vi "TRAJECTORY_EXECUTE_SWERVE.vi"(4 "Time Offset":dbl=-1.0 format="%16.4f", 6 "EnableClosedLoop":bool=TRUE, 8 "Init":bool, 9 "Reverse":bool, 10 "Follow Orientation":bool, 11 "Gyro Heading\nRAD":dbl) -> (0 "AtReference":bool, 1 "OutputTRAJ_STATE":T6={"TimeSeconds"=0.0, "Velocity"=0.0, "Acceleration"=0.0, "POSE"={"TRANSLATION"={"X"=0.0, "Y"=0.0}, "ROTATION"={"VALUE"=0.0, "COS"=1.0, "SIN"=0.0}}, "Curvature"=0.0} {"POSE"."ROTATION"."SIN" format="%13.4f"; "POSE"."ROTATION"."COS" format="%13.4f"; "POSE"."ROTATION"."VALUE" format="%13.4f"; "POSE"."TRANSLATION"."Y" format="%14.3f"; "POSE"."TRANSLATION"."X" format="%14.3f"}, 2 "Error and Corr":T4 {"Error Pose"."ROTATION"."SIN" format="%13.4f"; "Error Pose"."ROTATION"."COS" format="%13.4f"; "Error Pose"."ROTATION"."VALUE" format="%13.4f"; "Error Pose"."TRANSLATION"."Y" format="%14.3f"; "Error Pose"."TRANSLATION"."X" format="%14.3f"}, 3 "Chassis Velocity Target":T5 {"vOmega" format="%10.3f"; "vY" format="%10.3f"; "vX" format="%10.3f"}, 5 "Orientation Target":dbl)   [LabVIEW 2019]
uses:
  <vilib>/Rock Robotics/WPI/ThirdParty/JAS_Junk/TrajLib/TRAJ_STATE.ctl
  <vilib>/Rock Robotics/WPI/ThirdParty/JAS_Junk/TrajLib/POSE2D.ctl
  <vilib>/Rock Robotics/WPI/ThirdParty/JAS_Junk/TrajLib/TRANSLATION2D.ctl
  <vilib>/Rock Robotics/WPI/ThirdParty/JAS_Junk/TrajLib/ROTATION2D.ctl
  <vilib>/Rock Robotics/WPI/ThirdParty/JAS_Junk/TrajLib/CHASSIS_SPEEDS.ctl
  <vilib>/Rock Robotics/WPI/ThirdParty/JAS_Junk/TrajLib/Translation_Create.vi
  <vilib>/Rock Robotics/WPI/ThirdParty/JAS_Junk/TrajLib/ProfiledPIDController_NewPeriod.vi
  <vilib>/Rock Robotics/WPI/ThirdParty/JAS_Junk/TrajLib/PIDController_NewPeriod.vi
  <vilib>/Rock Robotics/WPI/ThirdParty/JAS_Junk/TrajLib/MathUtil_InputModulus.vi
  <vilib>/Rock Robotics/WPI/ThirdParty/JAS_Junk/TrajLib/Rotation_UnaryMinus.vi
  <vilib>/Rock Robotics/WPI/ThirdParty/JAS_Junk/TrajLib/Rotation_RotateBy.vi
  <vilib>/Rock Robotics/WPI/ThirdParty/JAS_Junk/TrajLib/HolDrvCtrl_Calculate.vi
  <vilib>/Rock Robotics/WPI/ThirdParty/JAS_Junk/TrajLib/Pose_getXYAngle.vi
  <vilib>/Rock Robotics/WPI/ThirdParty/JAS_Junk/TrajLib/TrapProfState_New.vi
  <vilib>/Rock Robotics/SystemInterfaces/NetworkCommunication/NetComm_UsageReport_report.vi
  <vilib>/Rock Robotics/WPI/ThirdParty/JAS_Junk/TrajLib/Rotation_CreateXY.vi
  <vilib>/Rock Robotics/WPI/ThirdParty/JAS_Junk/TrajLib/ProfiledPIDController_Calculate_Meas_Goal.vi
  <vilib>/Rock Robotics/WPI/ThirdParty/JAS_Junk/TrajLib/ChassisSpeeds_FromFieldRelativeSpeeds.vi
  <vilib>/Rock Robotics/WPI/ThirdParty/JAS_Junk/TrajLib/PIDController_Reset.vi
  <vilib>/Rock Robotics/WPI/ThirdParty/JAS_Junk/TrajLib/PIDController_Calculate_SP_PV.vi
  <vilib>/Rock Robotics/WPI/ThirdParty/JAS_Junk/TrajLib/ProfiledPIDController_Reset_PosOnly.vi
  <vilib>/Rock Robotics/WPI/ThirdParty/JAS_Junk/TrajLib/Rotation_GetAngleCosSin.vi
  <vilib>/Rock Robotics/WPI/ThirdParty/JAS_Junk/TrajLib/Pose_RelativeTo.vi
  <vilib>/Rock Robotics/WPI/ThirdParty/JAS_Junk/TrajLib/Util_CalcDist.vi
  <vilib>/Rock Robotics/WPI/ThirdParty/JAS_Junk/TrajLib/ProfiledPIDController_SetGoal_PosOnly.vi
  <vilib>/Rock Robotics/WPI/ThirdParty/JAS_Junk/TrajLib/ProfiledPIDController_Calculate_Meas.vi
  <vilib>/Rock Robotics/WPI/ThirdParty/JAS_Junk/TrajLib/Rotation_GetCos.vi
  <vilib>/Rock Robotics/WPI/ThirdParty/JAS_Junk/TrajLib/Rotation_GetSin.vi
  <vilib>/Rock Robotics/WPI/ThirdParty/JAS_Junk/TrajLib/PIDController_SetSetpoint.vi
  <vilib>/Rock Robotics/WPI/ThirdParty/JAS_Junk/TrajLib/PIDController_Calculate_PV.vi
  <vilib>/Rock Robotics/WPI/ThirdParty/JAS_Junk/TrajLib/ProfiledPIDController_Reset.vi
  <vilib>/Rock Robotics/WPI/ThirdParty/JAS_Junk/TrajLib/Transform_Create_PosePose.vi
  <vilib>/Rock Robotics/WPI/ThirdParty/JAS_Junk/TrajLib/ProfiledPIDController_SetGoal.vi
  <vilib>/Rock Robotics/WPI/ThirdParty/JAS_Junk/TrajLib/TrapProfile_New.vi
  <vilib>/Rock Robotics/WPI/ThirdParty/JAS_Junk/TrajLib/ProfiledPIDController_GetPeriod.vi
  <vilib>/Rock Robotics/WPI/ThirdParty/JAS_Junk/TrajLib/TrapProfile_Calculate.vi
  <vilib>/Rock Robotics/WPI/ThirdParty/JAS_Junk/TrajLib/ControllerUtil_GetModulusError.vi
  <vilib>/Rock Robotics/WPI/ThirdParty/JAS_Junk/TrajLib/Translation_RotateBy.vi
  <vilib>/Rock Robotics/WPI/ThirdParty/JAS_Junk/TrajLib/Translation_Minus.vi
  <vilib>/Rock Robotics/WPI/ThirdParty/JAS_Junk/TrajLib/TrapProfile_ShouldFlipAcceleration.vi
  <vilib>/Rock Robotics/WPI/ThirdParty/JAS_Junk/TrajLib/TrapProfile_Direct.vi
  <vilib>/Rock Robotics/WPI/ThirdParty/JAS_Junk/TrajLib/PIDController_GetPeriod.vi
  <vilib>/Rock Robotics/WPI/ThirdParty/JAS_Junk/TrajLib/Util_LibraryGlobals.vi
  <vilib>/Rock Robotics/WPI/ThirdParty/JAS_Junk/TrajLib/Trajectory_Library.lvlib
panel:
  # "(FOR TESTING)"
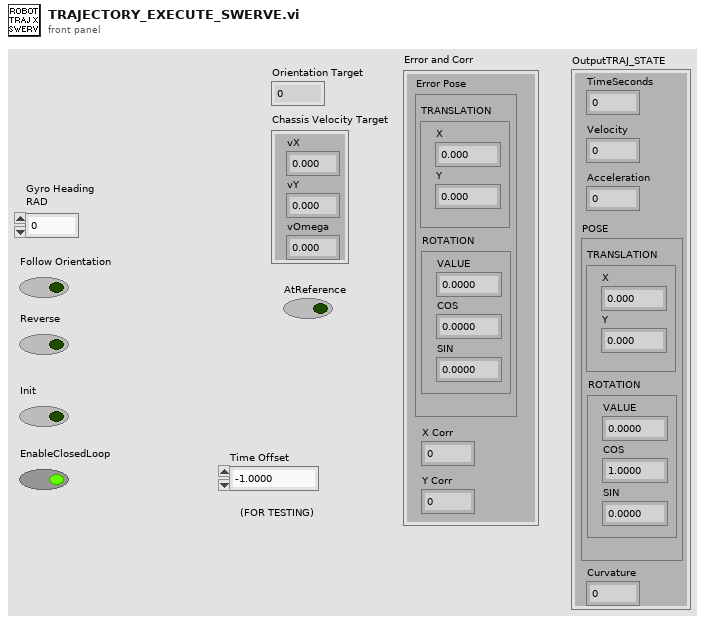
[diagram p1: front panel]
types:
  T1 = typedef "Trajectory_Library.lvlib/POSE2D.ctl" = cluster{"TRANSLATION":T2, "ROTATION":T3}
  T2 = typedef "Trajectory_Library.lvlib/TRANSLATION2D.ctl" = cluster{"X":dbl, "Y":dbl}
  T3 = typedef "Trajectory_Library.lvlib/ROTATION2D.ctl" = cluster{"VALUE":dbl, "COS":dbl, "SIN":dbl}
  T4 = cluster{"Error Pose":T1, "X Corr":dbl, "Y Corr":dbl}
  T5 = typedef "Trajectory_Library.lvlib/CHASSIS_SPEEDS.ctl" = cluster{"vX":dbl, "vY":dbl, "vOmega":dbl}
  T6 = typedef "Trajectory_Library.lvlib/TRAJ_STATE.ctl" = cluster{"TimeSeconds":dbl, "Velocity":dbl, "Acceleration":dbl, "POSE":T1, "Curvature":dbl}
  T7 = typedef "Trajectory_Library.lvlib/SWERVE_DRIVE_KINEMATICS.ctl" = cluster{"NumModules":i32, "InverseKinematics":T8, "ForwardKinematics":T8, "Modules":T2[], "PrevCoR":T2}
  T8 = typedef "NI_Matrix.lvlib/RealMatrix.ctl" = dbl[][]
  T9 = typedef "Trajectory_Library.lvlib/SWERVE_DRIVE_ODOMETRY.ctl" = cluster{"POSE":T1, "GyroOffset":T3, "PreviousAngle":T3, "PrevTime":dbl}
  T10 = typedef "Trajectory_Library.lvlib/TRAJECTORY.ctl" = cluster{"TotalTImeSecs":dbl, "States":T6[]}
  T11 = typedef "Trajectory_Library.lvlib/SWERVE_DRIVE_MODULE_STATE.ctl" = cluster{"Speed":dbl, "Angle":T3}
  T12 = typedef "Trajectory_Library.lvlib/PID_TUNING.ctl" = cluster{"Kp":dbl, "Ki":dbl, "Kd":dbl, "MaximumIntegral":dbl, "MinimumIntegral":dbl}
  T13 = typedef "Trajectory_Library.lvlib/PROFILED_PID_CONTROLLER.ctl" = cluster{"Controller":T14, "Goal":T15, "Setpoint":T15, "Constraint":T16}
  T14 = typedef "Trajectory_Library.lvlib/PID_CONTROLLER.ctl" = cluster{"Kp":dbl, "Ki":dbl, "Kd":dbl, "Period":dbl, "Max_Integral":dbl, "Min_Integral":dbl, "Max_Input":dbl, "Min_Input":dbl, "Continuous":bool, "PositionError":dbl, "VelocityError":dbl, "PrevError":dbl, "TotalError":dbl, "PositionTolerance":dbl, "VelocityTolerance":dbl, "SetPoint":dbl, "Kf":dbl, "Prev_Deriv":dbl, "Prev_Deriv 2":dbl, "DerivativeFilter":bool, "Min_Output":dbl, "Max_Output":dbl, "Prev_F_P":dbl, "Prev_F_P_2":dbl, "AntiWindupActive":bool, "Measurement":dbl}
  T15 = typedef "Trajectory_Library.lvlib/TRAPEZOID_PROFILE_STATE.ctl" = cluster{"Position":dbl, "Velocity":dbl}
  T16 = typedef "Trajectory_Library.lvlib/TRAPEZOID_PROFILE_CONSTRAINT.ctl" = cluster{"MaxVelocity":dbl, "MaxAcceleration":dbl}
  T17 = typedef "Trajectory_Library.lvlib/HOLONOMIC_DRV_CTRL.ctl" = cluster{"poseTolerance":T1, "poseError":T1, "Enabled":bool, "PID_xCtrl":T14, "PID_yCtrl":T14, "PROF_PID_thetaCtrl":T13, "RotationError":T3, "FirstRun":bool}
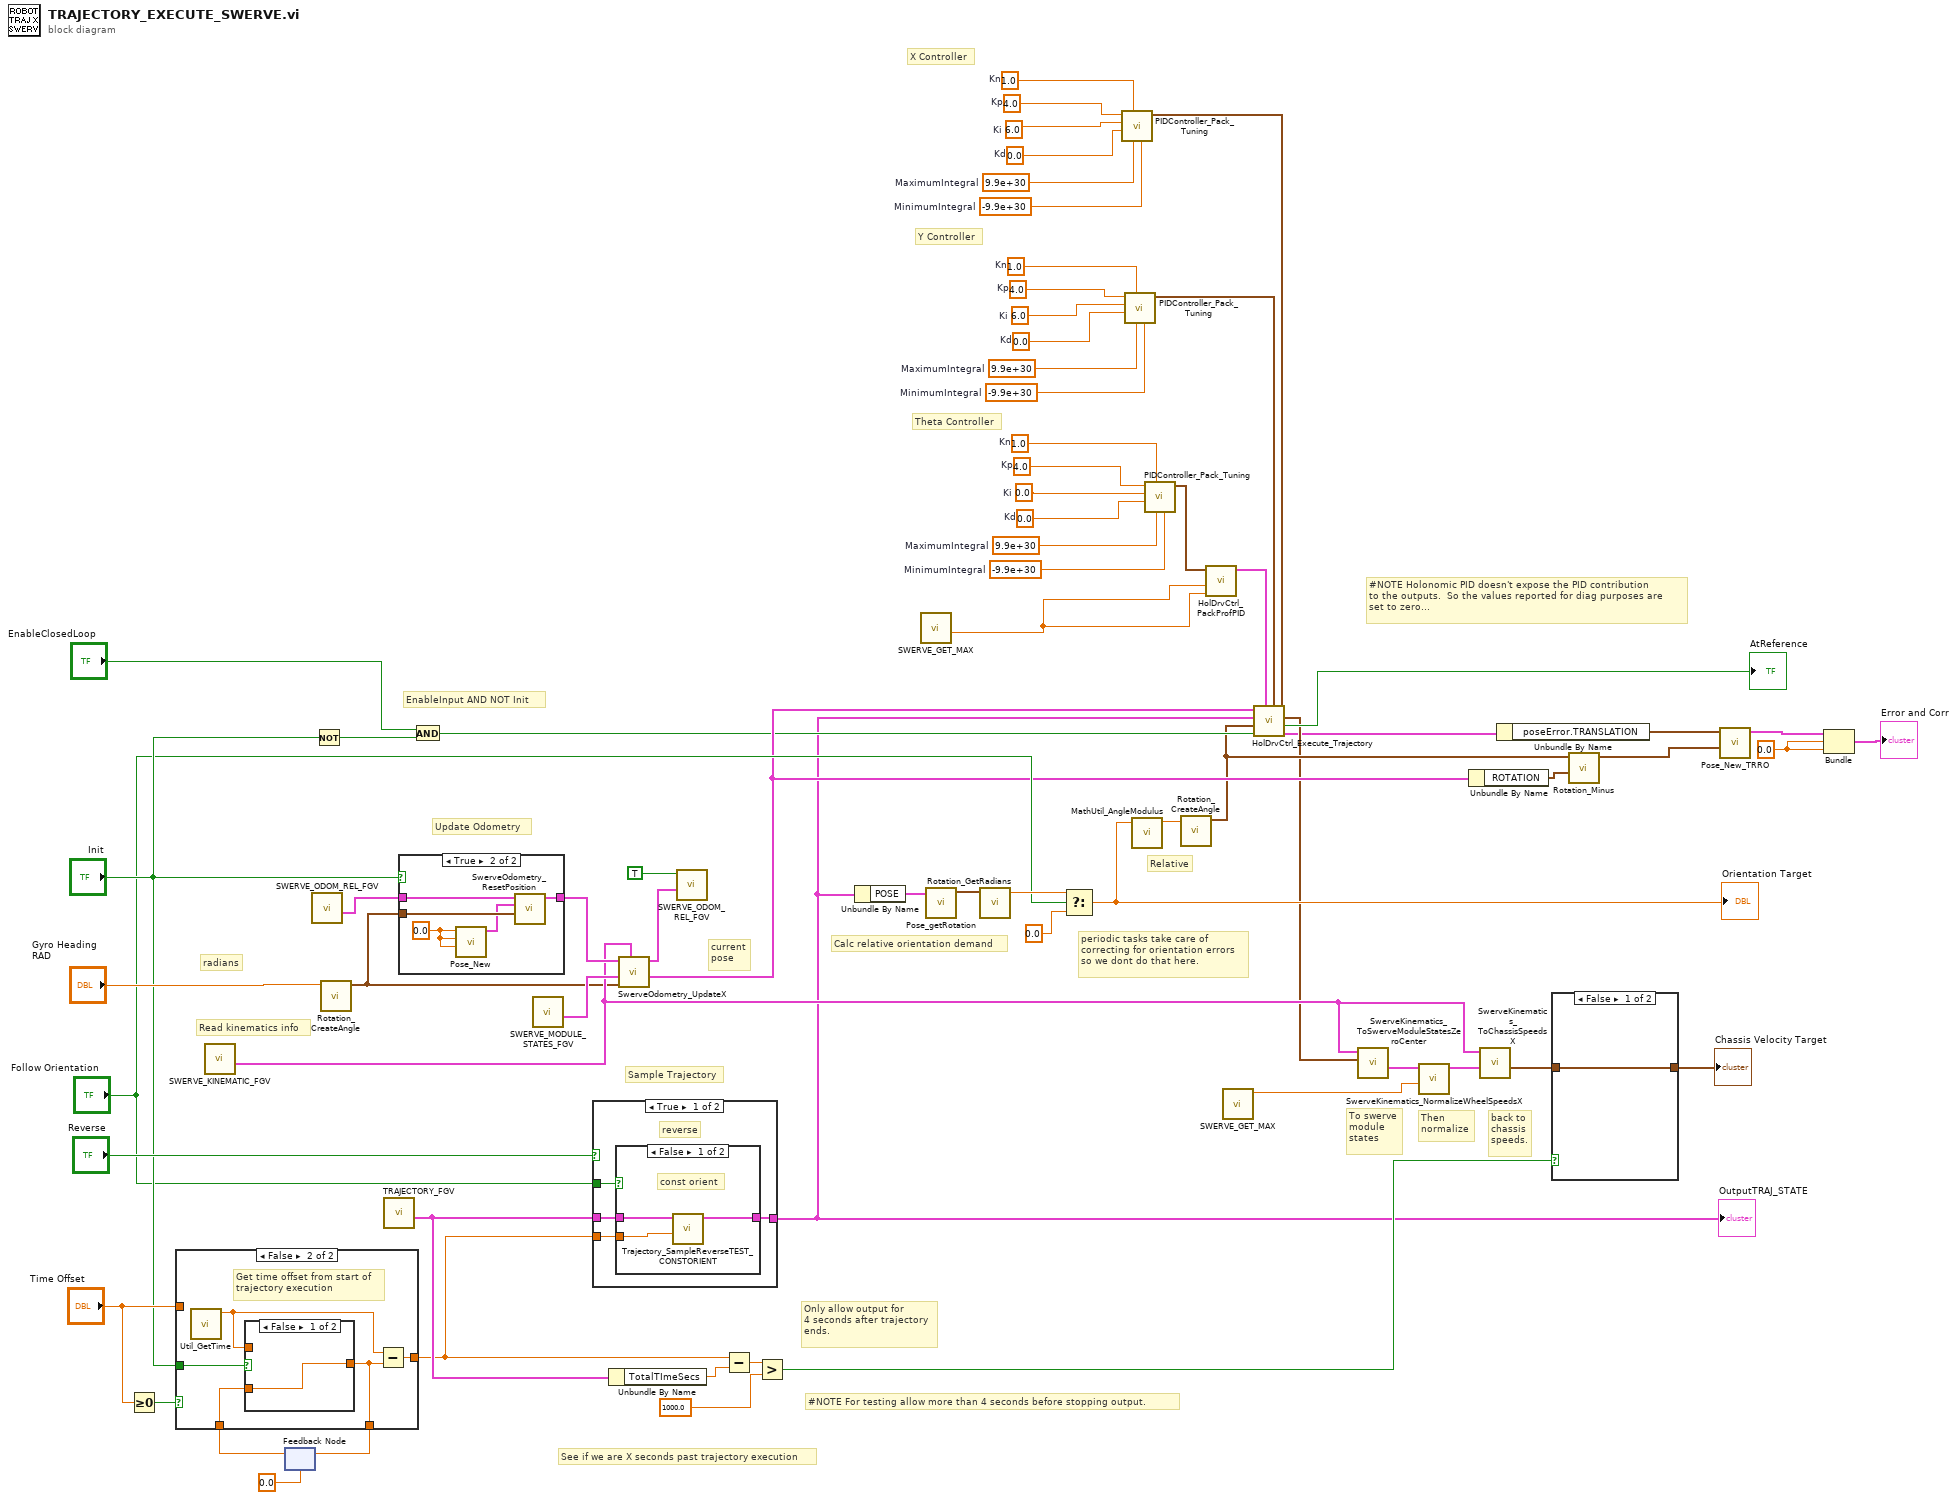
[diagram p0: block diagram]
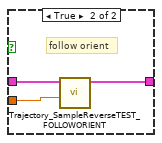
[diagram p4: hidden frame]
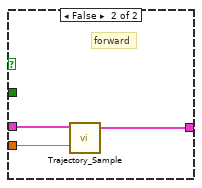
[diagram p5: hidden frame]
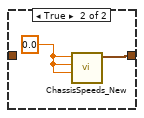
[diagram p7: hidden frame]
diagram:
  w15 = 1.0  # Kn
  w18 = 4.0  # Kp
  w27 = 0.0  # Ki
  w28 = 0.0  # Kd
  w29 = 9.9e+30  # MaximumIntegral
  w30 = -9.9e+30  # MinimumIntegral
  w13 = 1.0  # Kn
  w16 = 4.0  # Kp
  w19 = 6.0  # Ki
  w20 = 0.0  # Kd
  w21 = 9.9e+30  # MaximumIntegral
  w22 = -9.9e+30  # MinimumIntegral
  w14 = 1.0  # Kn
  w17 = 4.0  # Kp
  w23 = 6.0  # Ki
  w24 = 0.0  # Kd
  w25 = 9.9e+30  # MaximumIntegral
  w26 = -9.9e+30  # MinimumIntegral
  w43 = 0.0
  # "#NOTE For testing allow more than 4 seconds before stopping output."
  # "EnableInput AND NOT Init"
  # "Theta Controller"
  # "Y Controller"
  # "X Controller"
  # "Relative"
  # "#NOTE Holonomic PID doesn't expose the PID contribution \nto the outputs.  So the values reported for diag purposes are\nset to zero..."
  # "current\npose"
  # "back to\nchassis\nspeeds."
  # "Then\nnormalize"
  # "To swerve\nmodule\nstates"
  # "Calc relative orientation demand"
  # "Read kinematics info"
  # "Sample Trajectory"
  # "See if we are X seconds past trajectory execution"
  # "Update Odometry"
  # "radians"
  # "periodic tasks take care of\ncorrecting for orientation errors\nso we dont do that here."
  # "Only allow output for\n4 seconds after trajectory\nends."
  n1 = Greater Or Equal To 0?(x="Time Offset") -> (x >= 0?=w47:bool)
  n2 = call "SWERVE_KINEMATIC_FGV.vi"() -> ("out SWERVE_DRIVE_KINEMATICS"=w58:T7)  [unwired: 11 in]
  n3 = feedback #1(0.0 ("TIME")) -> (w49:dbl)
  n4 = case shown="False" w47 {
    tunnel: [w72 w78] -> w69
    tunnel: "Init" -> [_ w76]
    tunnel: w49 -> [w73 w75]
    tunnel: [w73 w74] -> w48
    tunnel: "Time Offset" -> [w72 _]
    frame True {
      # "For testing allow\nuser entered time offset!!"
    }
    frame False {
      # "Get time offset from start of\ntrajectory execution"
      n5 = call <vilib>:"Util_GetTime.vi"() -> ("FPGA_Time_Seconds"=w77:dbl)  [unwired: 10 in, 1 out]
      n6 = case shown="False" w76 {
        tunnel: [w79 w80] -> w74
        tunnel: w75 -> [w79 _]
        tunnel: w77 -> [_ w80]
        frame False {
        }
        frame True {
        }
      }
      n7 = Subtract(x=w77, y=w74) -> (x-y=w78:dbl)
    }
  }
  n8 = feedback-in #1(w48) -> ()
  n9 = call "SWERVE_ODOM_REL_FGV.vi"() -> ("out SWERVE_DRIVE_ODOMETRY"=w64:T9)  [unwired: 11 in]
  n10 = Not(x="Init") -> (.not. x?=w44:bool)
  n11 = call <vilib>:"Rotation_CreateAngle.vi"("Angle"="Gyro Heading\nRAD") -> ("ROTATION"=w39:T3)  [unwired: 10 in]
  n12 = call "TRAJECTORY_FGV.vi"() -> ("outTRAJECTORY"=w71:T10)  [unwired: 11 in]
  n13 = case shown="True" "Init" {
    tunnel: w64 -> [w81 w86]
    tunnel: [w81 w85] -> w63
    tunnel: w39 -> [_ w84]
    frame False {
    }
    frame True {
      w83 = 0.0 ("X")
      n14 = call <vilib>:"Pose_New.vi"("Heading"=w83, "Y"=w83, "X"=w83) -> ("out POSe"=w82:T1)  [unwired: 8 in]
      n15 = call <vilib>:"SwerveOdometry_ResetPosition.vi"("gyroAngle"=w84, "Pose"=w82, "in SWERVE_DRIVE_ODOMETRY"=w86) -> ("out SWERVE_DRIVE_ODOMETRY"=w85:T9)  [unwired: 8 in]
    }
  }
  n16 = And(x="EnableClosedLoop", y=w44) -> (x .and. y?=w6:bool)
  n17 = call "SWERVE_MODULE_STATES_FGV.vi"() -> ("out Current Module States"=w61:T11[])  [unwired: 11 in]
  n18 = case shown="True" "Reverse" {
    tunnel: w71 -> [w90 w99]
    tunnel: w69 -> [w88 w98]
    tunnel: [w89 w97] -> w5
    tunnel: "Follow Orientation" -> [w87 _]
    frame True {
      # "reverse"
      n19 = case shown="False" w87 {
        tunnel: w90 -> [w93 w96]
        tunnel: [w91 w95] -> w89
        tunnel: w88 -> [w92 w94]
        frame False {
          # "const orient"
          n20 = call "Trajectory_SampleReverseTEST_CONSTORIENT.vi"("Time"=w92, "InputTRAJECTORY"=w93) -> ("OutputTRAJ_STATE"=w91:T6)  [unwired: 9 in]
        }
        frame True {
          # "follow orient"
          n21 = call "Trajectory_SampleReverseTEST_FOLLOWORIENT.vi"("Time"=w94, "InputTRAJECTORY"=w96) -> ("OutputTRAJ_STATE"=w95:T6)  [unwired: 9 in]
        }
      }
    }
    frame False {
      # "forward"
      n22 = call <vilib>:"Trajectory_Sample.vi"("Time"=w98, "InputTRAJECTORY"=w99) -> ("OutputTRAJ_STATE"=w97:T6)  [unwired: 9 in]
    }
  }
  "OutputTRAJ_STATE" <- w5
  n23 = Unbundle By Name(w71) -> ("TotalTImeSecs"=w70:dbl)
  n24 = call <vilib>:"SwerveOdometry_UpdateX.vi"("SWERVE_DRIVE_KINEMATICS"=w58, "gyroAngle"=w39, "module States"=w61, "in SWERVE_DRIVE_ODOMETRY"=w63) -> ("robot POSE"=w7:T1, "out SWERVE_DRIVE_ODOMETRY"=w55:T9)  [unwired: 6 in]
  n25 = call "SWERVE_ODOM_REL_FGV.vi"("in SWERVE_DRIVE_ODOMETRY"=w55, "WRITE"=TRUE) -> ()  [unwired: 9 in, 1 out]
  n26 = Subtract(x=w69, y=w70) -> (x-y=w68:dbl)
  n27 = Greater?(x=w68, y=1000.0) -> (0:w66:bool)
  n28 = Unbundle By Name(w5) -> ("POSE"=w51:T1)
  n29 = call "SWERVE_GET_MAX.vi"() -> ("Max Rotational Vel (Rad/Sec)"=w8:dbl)  [unwired: 10 in, 1 out]
  n30 = call <vilib>:"Pose_getRotation.vi"("in POSE"=w51) -> ("out ROTATION"=w57:T3)  [unwired: 10 in]
  n31 = call <vilib>:"Rotation_GetRadians.vi"("in ROTATION"=w57) -> ("AngleRadians"=w34:dbl)  [unwired: 10 in]
  n32 = Select(t=w34, s="Follow Orientation", f=0.0) -> (s? t:f=w31:dbl)
  "Orientation Target" <- w31
  n33 = call <vilib>:"PIDController_Pack_Tuning.vi"("MinimumIntegral"=w22, "MaximumIntegral"=w21, "Kn"=w13, "Kd"=w20, "Ki"=w19, "Kp"=w16) -> ("PID Tuning"=w9:T12)  [unwired: 5 in]
  n34 = call <vilib>:"PIDController_Pack_Tuning.vi"("MinimumIntegral"=w26, "MaximumIntegral"=w25, "Kn"=w14, "Kd"=w24, "Ki"=w23, "Kp"=w17) -> ("PID Tuning"=w10:T12)  [unwired: 5 in]
  n35 = call <vilib>:"MathUtil_AngleModulus.vi"("InputAngle"=w31) -> ("ModulsAngle"=w41:dbl)  [unwired: 10 in]
  n36 = call <vilib>:"PIDController_Pack_Tuning.vi"("MinimumIntegral"=w30, "MaximumIntegral"=w29, "Kn"=w15, "Kd"=w28, "Ki"=w27, "Kp"=w18) -> ("PID Tuning"=w12:T12)  [unwired: 5 in]
  n37 = call <vilib>:"Rotation_CreateAngle.vi"("Angle"=w41) -> ("ROTATION"=w4:T3)  [unwired: 10 in]
  n38 = call <vilib>:"HolDrvCtrl_PackProfPID.vi"("Max Accel"=w8, "Max Speed"=w8, "Theta PID Tuning"=w12) -> ("Theta PID CONTROLLER"=w11:T13)  [unwired: 8 in]
  n39 = call "SWERVE_GET_MAX.vi"() -> ("Max Wheel Vel (Meter/Sec)"=w52:dbl)  [unwired: 10 in, 1 out]
  n40 = call <vilib>:"HolDrvCtrl_Execute_Trajectory.vi"("X PID Tuning"=w9, "Y PID Tuning"=w10, "thetaProfiledPID_CTRL"=w11, "Enable"=w6, "angleRef"=w4, "desiredTrajState"=w5, "currentPose"=w7) -> ("outHOLONOMIC_DRV_CTRL"=w1:T17, "AtReference"=→"AtReference":bool, "calcChassisSpeed"=w2:T5)  [unwired: 2 in]
  n41 = call <vilib>:"SwerveKinematics_ToSwerveModuleStatesZeroCenter.vi"("ChassisSpeeds"=w2, "in SWERVE_DRIVE_KINEMATICS"=w58) -> ("ModuleStates"=w60:T11[])  [unwired: 8 in, 1 out]
  n42 = call <vilib>:"SwerveKinematics_NormalizeWheelSpeedsX.vi"("AttainableMaxSpeed"=w52, "in WheelStates"=w60) -> ("out WheelStates"=w59:T11[])  [unwired: 9 in]
  n43 = Unbundle By Name(w7) -> ("ROTATION"=w35:T3)
  n44 = call <vilib>:"SwerveKinematics_ToChassisSpeedsX.vi"("WheelStates"=w59, "in SWERVE_DRIVE_KINEMATICS"=w58) -> ("Chassis Speed"=w54:T5)  [unwired: 9 in]
  n45 = Unbundle By Name(w1) -> ("poseError.TRANSLATION"=w40:T2)
  n46 = case shown="False" w66 {
    tunnel: w54 -> [w100 _]
    tunnel: [w100 w101] -> w53
    frame False {
    }
    frame True {
      w102 = 0.0 ("vX")
      n47 = call <vilib>:"ChassisSpeeds_New.vi"("vAngular"=w102, "vY"=w102, "vX"=w102) -> ("CHASSIS"=w101:T5)  [unwired: 8 in]
    }
  }
  "Chassis Velocity Target" <- w53
  n48 = call <vilib>:"Rotation_Minus.vi"("other ROTATION"=w35, "in ROTATION"=w4) -> ("out ROTATION"=w38:T3)  [unwired: 9 in]
  n49 = call <vilib>:"Pose_New_TRRO.vi"("ROTATION"=w38, "TRANSLATION"=w40) -> ("outPOSE"=w37:T1)  [unwired: 9 in]
  n50 = Bundle("outPOSE"=w37, w43, w43) -> (→"Error and Corr":cluster{"outPOSE":T1, dbl, dbl})  [unwired: 1 in]
